vi "MIC Calculation.vi"() -> ()   [LabVIEW 2014]
panel:
  out "x-y":u32
  in  "Captured MIC":u8[](array[numeric])=[0, 0, 0, 0, 0, 0, 0, 0, 0, 0, 0, 0, 0, 0, 0, 0]
  out "x = y?":bool[](array[boolean])
  in  "Concatenated AP and STA info":u8[](array[numeric])=[0, 0, 0, 0, 0, 0, 0, 0, 0, 0, 0, 0, 0, 0, 0, 0, 0, 0, 0, 0, 0, 0, 0, 0, 0, 0, 0, 0, 0, 0, 0, 0, 0, 0, 0, 0, 0, 0, 0, 0, 0, 0, 0, 0, 0, 0, 0, 0, 0, 0, 0, 0, 0, 0, 0, 0, 0, 0, 0, 0, 0, 0, 0, 0, 0, 0, 0, 0, 0, 0, 0, 0, 0, 0, 0, 0, 0, 0, 0, 0, 0, 0, 0, 0, 0, 0, 0, 0, 0, 0, 0, 0, 0, 0, 0, 0, 0, 0, 0, 0]
  in  "Data":u8[](array[numeric])=[1, 0, 0, 0, 0, 0, 0, 0, 0, 0, 0, 0, 0, 0, 0, 0, 0, 0, 0, 0, 0, 0, 0, 0, 0, 0, 0, 0, 0, 0, 0, 0, 0, 0, 0, 0, 0, 0, 0, 0, 0, 0, 0, 0, 0, 0, 0, 0, 0, 0, 0, 0, 0, 0, 0, 0, 0, 0, 0, 0, 0, 0, 0, 0, 0, 0, 0, 0, 0, 0, 0, 0, 0, 0, 0, 0, 0, 0, 0, 0, 0, 0, 0, 0, 0, 0, 0, 0, 0, 0, 0, 0, 0, 0, 0, 0, 0, 0, 0, 0, 0, 0, 0, 0, 0, 0, 0, 0, 0, 0, 0, 0, 0, 0, 0, 0, 0, 0, 0, 0, 0] format="%x"
  in  "SSID":u8[](array[numeric])=[0, 0, 0, 0, 0, 0]
  in  "Secret Key":u8[](array[numeric])=[0, 0, 0, 0, 0, 0, 0, 0, 0, 0]
  # "Captured MIC: 932c83c6ee03041ac6c838167e4ef2a0"
  # "Note: The MIC comes from Frame 2 of EAPOL Packets.\n\nAlso take the Data under 802.1X-2001 from Packet 2, remove the MIC\nfrom it  and enter it in as data"
  # "Need to change length of SSID \nbecause this can change"
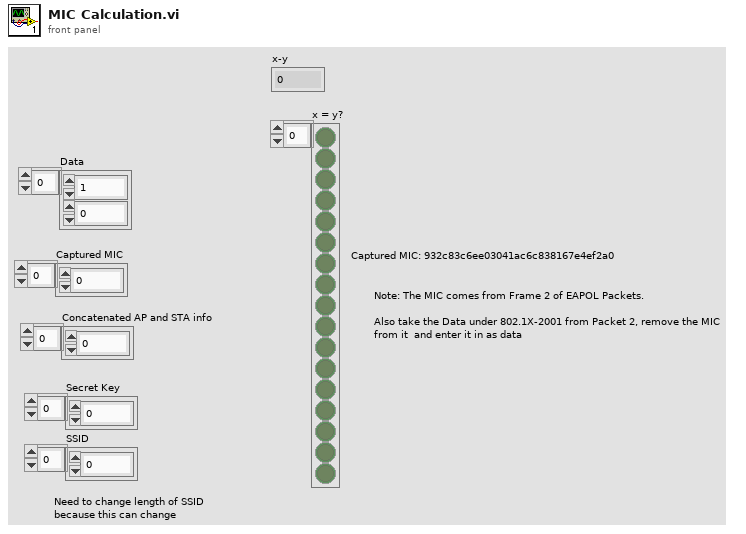
[diagram p1: front panel]
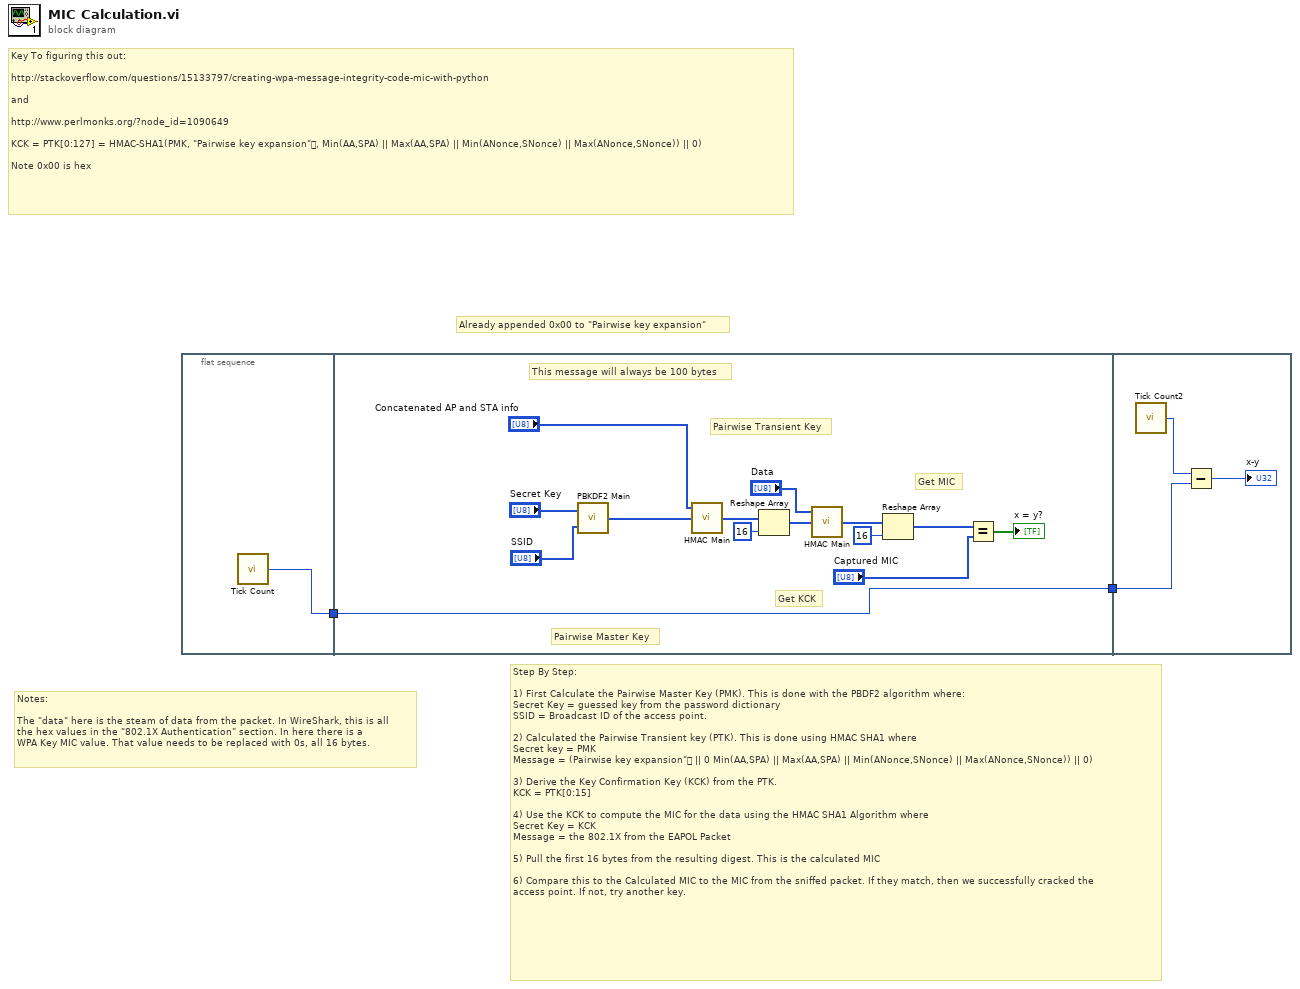
[diagram p0: block diagram]
diagram:
  # "Step By Step:\n\n1) First Calculate the Pairwise Master Key (PMK). This is done with the PBDF2 algorithm where:\nSecret Key = guessed key from the password dictionary\nSSID = Broadcast ID of the access point.\n\n2) Calculated the Pairwise Transient key (PTK). This is done using HMAC SHA1 where\nSecret key = PMK\nMessage = (Pairwise key expansion\" || 0 Min(AA,SPA) || Max(AA,SPA) || Min(ANonce,SNonce) || Max(ANonce,SNonce)) || 0) \n\n3) Derive the Key Confirmation Key (KCK) from the PTK. \nKCK = PTK[0:15]\n\n4) Use the KCK to compute the MIC for the data using the HMAC SHA1 Algorithm where\nSecret Key = KCK\nMessage = the 802.1X from the EAPOL Packet\n\n5) Pull the first 16 bytes from the resulting digest. This is the calculated MIC\n\n6) Compare this to the Calculated MIC to the MIC from the sniffed packet. If they match, then we successfully cracked the \naccess point. If not, try another key."
  # "Already appended 0x00 to \"Pairwise key expansion\""
  # "Notes:\n\nThe \"data\" here is the steam of data from the packet. In WireShark, this is all\nthe hex values in the \"802.1X Authentication\" section. In here there is a \nWPA Key MIC value. That value needs to be replaced with 0s, all 16 bytes."
  # "Key To figuring this out:\n\nhttp://stackoverflow.com/questions/15133797/creating-wpa-message-integrity-code-mic-with-python\n\nand\n\nhttp://www.perlmonks.org/?node_id=1090649\n\nKCK = PTK[0:127] = HMAC-SHA1(PMK, \"Pairwise key expansion\", Min(AA,SPA) || Max(AA,SPA) || Min(ANonce,SNonce) || Max(ANonce,SNonce)) || 0)\n\nNote 0x00 is hex"
  n1 = flat-sequence {
    tunnel: [w3] -> w1
    tunnel: [w4] -> w2
    tunnel: w1 -> [w4]
    tunnel: w2 -> [w19]
    frame #0 {
      n2 = call "Tick Count"() -> ("Tick Count(Ticks)"=w3:u32)
    }
    frame #1 {
      # "Pairwise Master Key"
      # "Get MIC"
      # "Get KCK"
      # "This message will always be 100 bytes"
      # "Pairwise Transient Key"
      n3 = call "PBKDF2 Main.vi"("SSID"="SSID", "Secret Key"="Secret Key") -> ("PSK"=w12:u8[])
      n4 = call "HMAC Main.vi"("Secret Key"=w12, "Message"="Concatenated AP and STA info") -> ("HMAC Out"=w15:u8[])  [unwired: 1 in]
      n5 = Reshape Array(w15, 16 ("dimension size")) -> (w13:u8[])
      n6 = call "HMAC Main.vi"("Secret Key"=w13, "Message"="Data") -> ("HMAC Out"=w17:u8[])  [unwired: 1 in]
      n7 = Reshape Array(w17, 16 ("dimension size")) -> (w9:u8[])
      n8 = Equal?(x=w9, y="Captured MIC") -> (x = y?=→"x = y?":bool[])
    }
    frame #2 {
      n9 = call "Tick Count2"() -> ("Tick Count(Ticks)"=w20:u32)
      n10 = Subtract(x=w20, y=w19) -> (x-y=→"x-y":u32)
    }
  }
